vi "ADXL345 SPI Accelerometer.vi"() -> ()   [LabVIEW 2025]
doc: "ADXL345 SPI Accelerometer\n\nThis example shows how to use the ADXL 345 Accelerometer sensor connected to SPI.\n\nThis example expects a USB cable connected from your development PC to the Type B USB Jack (next to the power input) on the roboRIO."
uses:
  <vilib>/Rock Robotics/SystemInterfaces/spilib/spi_bus.ctl
  <vilib>/Rock Robotics/WPI/Accelerometer/ADXL345 Range.ctl
  <vilib>/Rock Robotics/WPI/Accelerometer/WPI_AccelerometerADXL345 Axes.ctl
  <vilib>/Rock Robotics/WPI/Accelerometer/WPI_AccelerometerADXL345_SPI_Open.vi
panel:
  out "Z Acceleration":dbl
  out "Y Acceleration":dbl
  in  "ADXL345 Axes":T1={"X-Axis"=TRUE, "Y-Axis"=FALSE, "Z-Axis"=FALSE}
  in  "Accel Range":T2 items=["+/- 2 g", "+/- 4 g", "+/- 8 g", "+/- 16 g"]
  in  "SPI Bus":T3=enum."SPI On-Board, CS1"
  out "X Acceleration":dbl
  out "error out":errorcluster
  in  "stop":bool
  # "Set these inputs before running."
  # "Output information"
  # "This shows wiring for the Analog Devices ADXL345 accelerometer."
  # "ADXL345\nCS (blue)--------\nDO (yellow)-----\nDI (green)-------\nCK (orange)-----\n5V (red)---------\n0V (black)-------"
  # "roboRIO\nSPI    CS1\nSPI    MISO\nSPI    MOSI\nSPI    SCLK\nSPI    5V\nSPI"
  # "accelerometer"
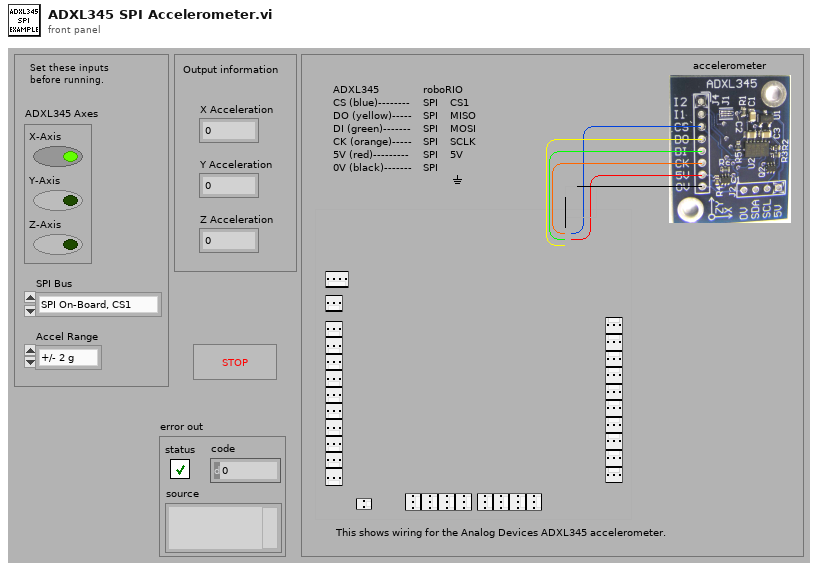
[diagram p1: front panel]
types:
  T1 = typedef "WPI_AccelerometerADXL345 Axes.ctl" = cluster{"X-Axis":bool, "Y-Axis":bool, "Z-Axis":bool}
  T2 = typedef "ADXL345 Range.ctl" = u8
  T3 = typedef "spi_bus.ctl" = enum16{"SPI On-Board, CS0", "SPI On-Board, CS1", "SPI On-Board, CS2", "SPI On-Board, CS3", "SPI MXP", "Invalid"}
  T4 = typedef "WPI_AccelerometerDevRef.ctl" = cluster{"DevStatus":errorcluster, "Scaling":T5, "Analog Channels":T6, "I2C Bus":T8, "SPI Bus":T3, "Accel Range":T2, "ADXL Axes":T1, "Handle":i32, "Device Address":u8, "Accel Type":enum16{"Analog", "ADXL345 I2C", "ADXL345 SPI", "Internal", "ADXL362 SPI"}}
  T5 = typedef "WPI_AccelerometerScaling.ctl" = cluster{"Gain (VoltsPerG)":dbl, "Center Voltage":dbl}
  T6 = typedef "WPI_AccelerometerAnalogChannels.ctl" = cluster{"X-Axis":T7, "Y-Axis":T7, "Z-Axis":T7}
  T7 = typedef "FPGA_AIChannel.ctl" = enum8{"AI 0", "AI 1", "AI 2", "AI 3", "AI MXP 0", "AI MXP 1", "AI MXP 2", "AI MXP 3", "Invalid"}
  T8 = typedef "i2c_bus.ctl" = enum16{"I2C On-Board", "I2C MXP", "Invalid"}
  T9 = cluster{"X-Axis":dbl, "Y-Axis":dbl, "Z-Axis":dbl}
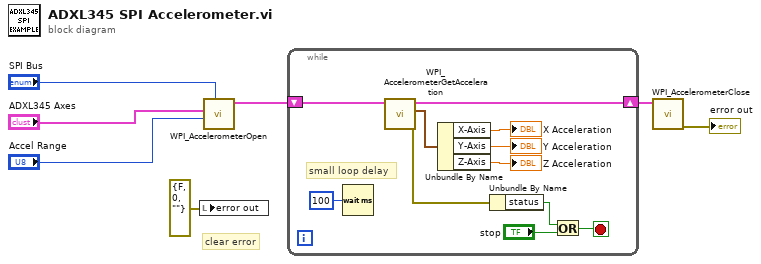
[diagram p0: block diagram]
diagram:
  # "clear error"
  n1 = local write "error out"(errorcluster {"status"=FALSE, "code"=0, "source"=""} ("error out")) -> ()
  n2 = call-poly <vilib>:"WPI_AccelerometerOpen.vi"("SPI Bus"="SPI Bus", "Accel Range"="Accel Range", "ADXL345 Axes"="ADXL345 Axes") -> ("AccelerometerDevRef"=w6:T4)  [unwired: 7 in, 1 out]
  n3 = while {
    shift-right: [w14] -> w2
    shift-left: w6 -> [w12]
    stop <- w13 stop-if-true
    # "small loop delay"
    n4 = Wait (ms)(milliseconds to wait=u32 100) -> ()  [unwired: 1 out]
    n5 = call <vilib>:"WPI_AccelerometerGetAcceleration.vi"("AccelerometerDevRef"=w12) -> ("error out"=w11:errorcluster, "Accelerations"=w15:T9, "AccelerometerDevRef"=w14:T4)  [unwired: 8 in]
    n6 = Unbundle By Name(w15) -> ("X-Axis"=→"X Acceleration":dbl, "Y-Axis"=→"Y Acceleration":dbl, "Z-Axis"=→"Z Acceleration":dbl)
    n7 = Unbundle By Name(w11) -> ("status"=w18:bool)
    n8 = Or(x=w18, y="stop") -> (x .or. y?=w13:bool)
  }
  n9 = call <vilib>:"WPI_AccelerometerClose.vi"("AccelerometerDevRef"=w2) -> ("error out"=→"error out":errorcluster)  [unwired: 10 in]
